vi "SVT Get Octave Subset.vi"   [LabVIEW 2017, in "SoundVib_Octave_2014 standard.lvlib"]
doc: "Extracts the subset of the <B>octave spectrum</B> specified by <B>frequency range</B> for a single channel or N channels. Wire data to the <B>octave spectrum</B> input to determine the polymorphic instance to use or manually select the instance."
uses:
  <vilib>/addons/Sound and Vibration/svt_Octave/SoundVib_Octave_2014 standard.lvlib
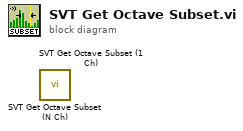
[diagram p0: block diagram]
diagram:
  n1 = call <vilib>:"SVT Get Octave Subset (N Ch).vi"() -> ()  [unwired: 11 in, 5 out]
  n2 = call <vilib>:"SVT Get Octave Subset (1 Ch).vi"() -> ()  [unwired: 11 in, 5 out]
